vi "Disconnect.vi"(8 "error in (no error)":errorcluster, 11 "PVConnection in":refnum<class "SVConnection.lvclass">) -> (0 "error out":errorcluster, 3 "PVConnection out":refnum<class "SVConnection.lvclass">)   [LabVIEW 2013, in "CS++ProcessVariables.lvlib" / "SVConnection.lvclass"]
doc: "Opene reference to a process variable."
uses:
  SVConnection.lvclass
  SVConnection.lvclass/SVConnection.ctl
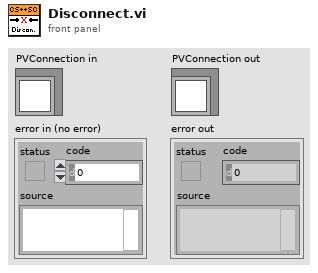
[diagram p1: front panel]
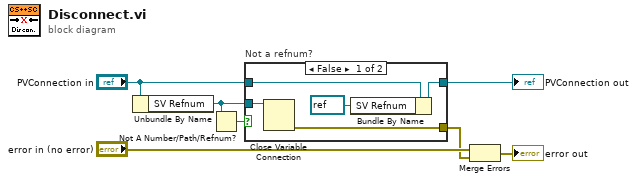
[diagram p0: block diagram]
diagram:
  n1 = Unbundle By Name("PVConnection in") -> ("SV Refnum"=w5:refnum<k21>)
  n2 = Not A Number/Path/Refnum?(number/path/refnum=w5) -> (NaN/Path/Refnum?=w4:bool)
  n3 = case "Not a refnum?" shown="False" w4 {
    tunnel: w5 -> [w12 _]
    tunnel: [w11 _] -> w1
    tunnel: "PVConnection in" -> [w10 w13]
    tunnel: [w9 w13] -> w6
    frame False {
      n4 = Close Variable Connection(11:w12) -> (0:w11:errorcluster)  [unwired: 1 in]
      n5 = Bundle By Name(cluster=w10, "SV Refnum"=refnum<k21> refnum) -> (w9:refnum<class "SVConnection.lvclass">)
    }
    frame True {
    }
  }
  "PVConnection out" <- w6
  n6 = Merge Errors("error in (no error)", w1) -> (→"error out":errorcluster)
